vi "EditNode.vi"(8 "Mouse Coords":T1={"Horizontal"=400, "Vertical"=400}, 11 "Node":refnum<k20>) -> ()   [LabVIEW 2019]
uses:
  <vilib>/Utility/miscctls.llb/LVPoint32TypeDef.ctl
  <resource>/objmgr/DOMUserDefRef.rc
panel:
  out "Array":string[][](array[string])
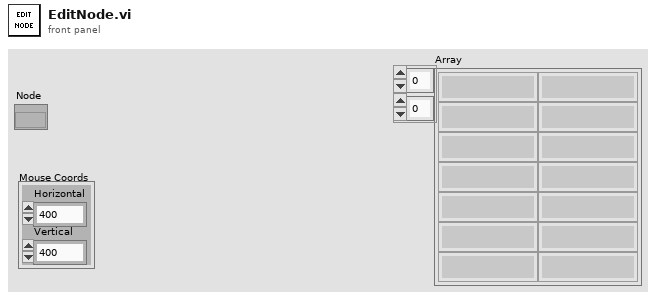
[diagram p1: front panel]
types:
  T1 = typedef "LVPoint32TypeDef.ctl" = cluster{"Horizontal":i32, "Vertical":i32}
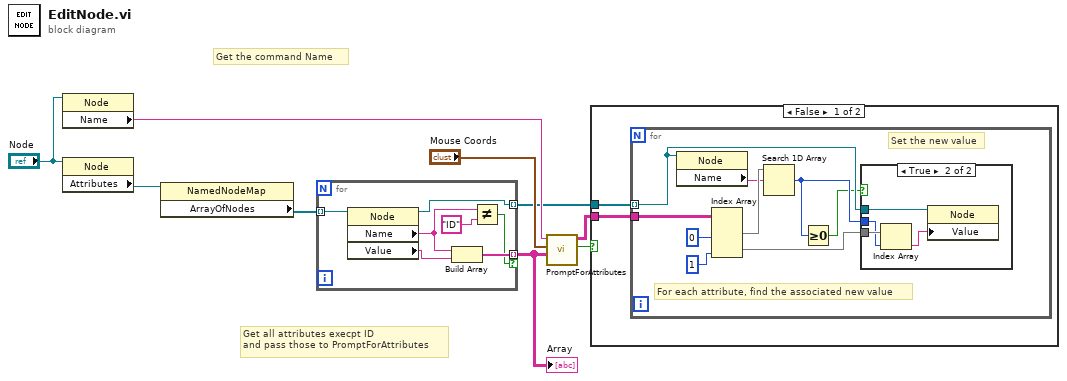
[diagram p0: block diagram]
diagram:
  # "Get all attributes execpt ID\nand pass those to PromptForAttributes"
  # "Get the command Name"
  n1 = property class="Node"(reference="Node") -> ("Name"=w6:string)  [unwired: 1 in, 2 out]
  n2 = property class="Node"(reference="Node") -> ("Attributes"=w9:refnum<k20>)  [unwired: 1 in, 2 out]
  n3 = property class="NamedNodeMap"(reference=w9) -> ("ArrayOfNodes"=w8:refnum<k20>[])  [unwired: 1 in, 2 out]
  n4 = for {
    tunnel: w8 -> [w14] mode=indexing
    tunnel: [w16] -> w1 mode=indexing if=w10
    tunnel: [w11] -> w4 mode=indexing
    n5 = property class="Node"(reference=w14) -> (reference out=w11:refnum<k20>, "Name"=w13:string, "Value"=w12:string)  [unwired: 1 in, 1 out]
    n6 = Build Array(w13, w12) -> (w16:string[])
    n7 = Not Equal?(x=w13, y="ID") -> (x != y?=w10:bool)
  }
  "Array" <- w1
  n8 = call "PromptForAttributes.vi"("Attributes In"=w1, "Mouse Coords"="Mouse Coords", "New Node Name"=w6) -> ("Canceled"=w2:bool, "Attributes"=w3:string[][])  [unwired: 7 in]
  n9 = case shown="False" w2 {
    tunnel: w4 -> [w18 _]
    tunnel: w3 -> [w17 _]
    frame False {
      n10 = for {
        tunnel: w18 -> [w24] mode=indexing
        tunnel: w17 -> [w25]
        # "Set the new value"
        # "For each attribute, find the associated new value"
        n11 = property class="Node"(reference=w24) -> ("Name"=w22:string)  [unwired: 1 in, 2 out]
        n12 = Index Array(array=w25, index (col) #1=0 ("disabled index (col)"), index (col) #2=1 ("index (col)")) -> (element #1=w23:string[], element #2=w21:string[])  [unwired: 2 in]
        n13 = Search 1D Array(1D array=w23, element=w22) -> (index of element=w20:i32)  [unwired: 1 in]
        n14 = Greater Or Equal To 0?(x=w20) -> (x >= 0?=w19:bool)
        n15 = case shown="True" w19 {
          tunnel: w24 -> [_ w31]
          tunnel: w21 -> [_ w30]
          tunnel: w20 -> [_ w28]
          frame False {
          }
          frame True {
            n16 = Index Array(array=w30, index=w28) -> (element=w29:string)
            n17 = property class="Node"(reference=w31, "Value"=w29) -> ()  [unwired: 1 in, 2 out]
          }
        }
      }
    }
    frame True {
      # "Canceled, don't modify"
    }
  }
